vi "HapticSPM_write.vi"() -> ()   [LabVIEW 2021]
uses:
  Haptic-Programming-Interface/LabVIEW VIs/Haptic Prog Interface/Haptic Prog Interface.lvlib
  <userlib>/Nanonis Prog Interface V5/Nanonis Prog Interface.lvlib
panel:
  out "Numeric 3":i32
  out "Numeric 2":i32
  out "Numeric":i32
  in  "Suggested Settings":bool=TRUE
  out "?":bool=TRUE
  out "Surface":dbl caption="Numeric" format="%#_2p"
  out "Z-Position":dbl caption="Numeric" format="%#_2p"
  out "y":string
  out "x":string
  out "scan data":dbl[][](array[numeric])
  out "Force":dbl(slide) scale=-3.0..3.0
  out "Frame String":string
  in  "Stop":bool
  out "Safe tip":bool
  out "Value":dbl caption="Numeric" format="%#_2p"
  out "Reframed Position (m)":cluster{"x (m)":dbl, "y (m)":dbl, "z (m)":dbl} {"z (m)" format="%.1p"; "y (m)" format="%.1p"; "x (m)" format="%.1p"}
  out "Frame Properties (m)":T1
  in  "Function":string(combo)="0" caption="Combo Box"
  in  "Gain (mm/pm)":dbl=1.0 caption="Numeric" format="%.1g"
  in  "k":dbl=1.0 caption="Numeric" step=0.1 format="%.1g"
  in  "Setpoint":dbl=1e-10 caption="Numeric" step=1e-11 format="%.0p"
  in  "Gain":dbl=1.0 caption="Numeric" format="%.1g"
  out "Click Number":dbl caption="Numeric" format="%#_1g"
  in  "Write Z":bool
  in  "Planing Toggle":bool
  in  "Planing Reset":bool
  in  "Save":bool
  # "Super Ultra Mega Haptic SPM Controller 3000"
  # "Scan Window"
  # "Height"
  # "Signal"
  # "Force"
  # "Force"
  # "Planing"
  # "Surface Scale"
  # "Move pens in all three dimensions to calibrate\nClick \"enter\" to turn off recommended settings"
  # "Z Write"
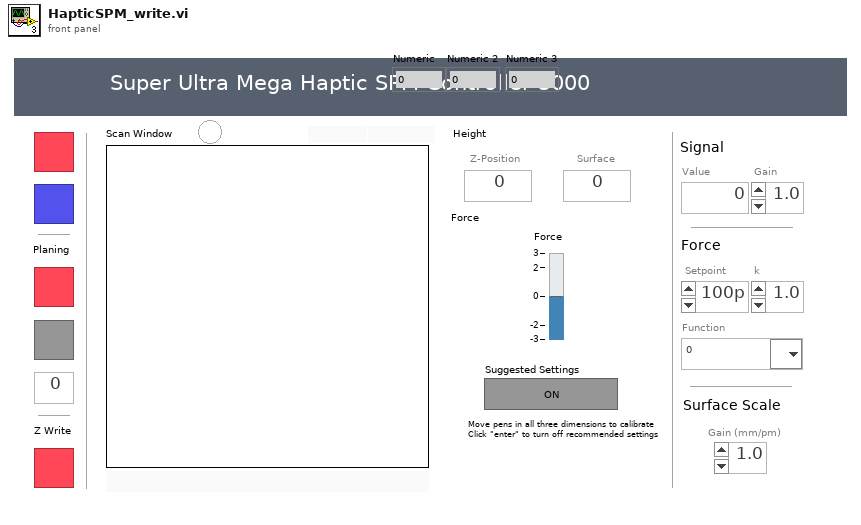
[diagram p1: front panel]
types:
  T1 = cluster{"Center coordinates (m)":cluster{"Xc":sgl, "Yc":sgl}, "Size (m)":cluster{"Width":sgl, "Height":sgl}}
  T2 = cluster{"Fx (N)":dbl, "Fy (N)":dbl, "Fz (N)":dbl}
  T3 = cluster{"kx (N/m)":dbl, "ky (N/m)":dbl, "kz (N/m)":dbl}
  T4 = cluster{"X Drag":bool, "Y Drag":bool, "Z Drag":bool}
  T5 = cluster{"Origin (m)":cluster{"X Origin (m)":dbl, "Y Origin (m)":dbl}, "Frame Size (m)":cluster{"FW (m)":dbl, "FH (m)":dbl}}
  T6 = cluster{"x (mm)":dbl, "y (mm)":dbl, "z (mm)":dbl}
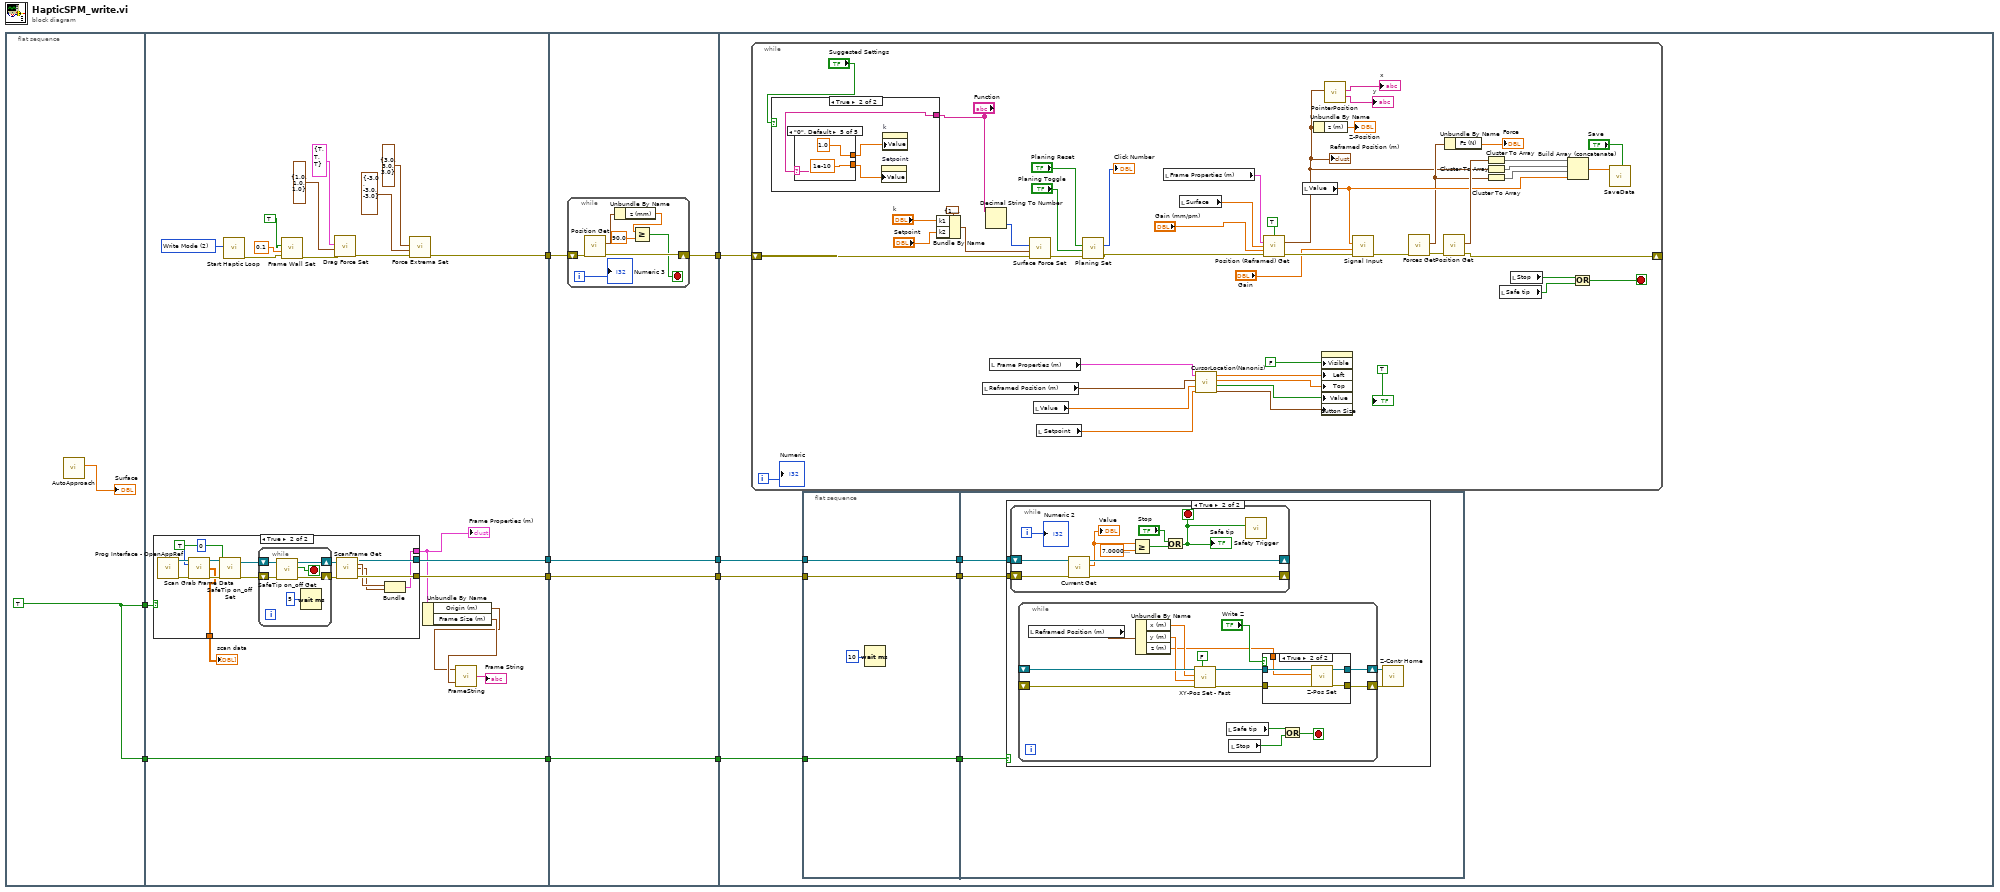
[diagram p0: block diagram]
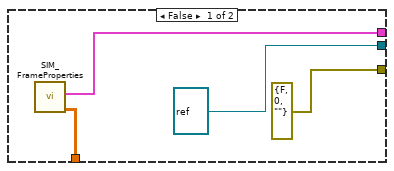
[diagram p2: hidden frame]
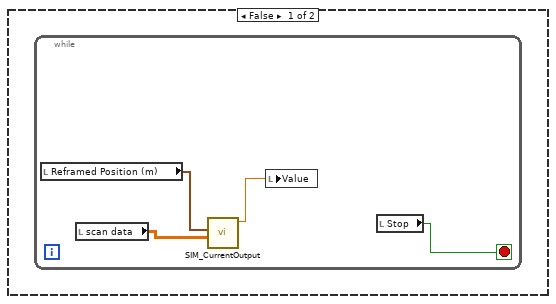
[diagram p3: hidden frame]
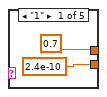
[diagram p6: hidden frame]
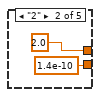
[diagram p7: hidden frame]
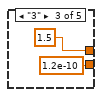
[diagram p8: hidden frame]
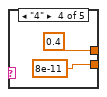
[diagram p9: hidden frame]
diagram:
  n1 = flat-sequence {
    tunnel: [w12] -> w4
    tunnel: [w12] -> w3
    tunnel: [w30] -> w10
    tunnel: [w21] -> w7
    tunnel: [w20] -> w5
    tunnel: w4 -> [w19]
    tunnel: w3 -> [w18]
    tunnel: [w18] -> w2
    tunnel: w10 -> [w63]
    tunnel: [w62] -> w9
    tunnel: [w61] -> w8
    tunnel: w7 -> [w61]
    tunnel: [w60] -> w6
    tunnel: w5 -> [w60]
    tunnel: w2 -> [w59]
    tunnel: [w59] -> w1
    tunnel: w9 -> [w77]
    tunnel: w8 -> [w75]
    tunnel: w6 -> [w73]
    tunnel: w1 -> [w72]
    frame #0 {
      w12 = TRUE
      n2 = call "AutoApproach.vi"() -> ("Surface Location (m)"=→"Surface":dbl)  [unwired: 11 in]
    }
    frame #1 {
      w32 = u16 2 items=["Custom Mode", "Read Mode", "Write Mode"] ("Mode Selection")
      n3 = case shown="True" w19 {
        tunnel: [refnum<vi> refnum ("Application ref out") w47] -> w21
        tunnel: [errorcluster {"status"=FALSE, "code"=0, "source"=""} ("error out") w46] -> w20
        tunnel: [w33 w37] -> w15
        tunnel: [w34 w41] -> w17
        frame False {
          n4 = call "SIM_FrameProperties.vi"() -> ("data"=w34:dbl[][], "Frame Properties (m)"=w33:T5)  [unwired: 9 in, 1 out]
        }
        frame True {
          n5 = call <userlib>:"Prog Interface - OpenAppRef.vi"() -> ("Error out"=w42:errorcluster, "Application reference"=w45:refnum<vi>)  [unwired: 6 in]
          n6 = call <userlib>:"Scan Grab Frame Data.vi"("Application ref in"=w45, "Channel index (0-23)"=u8 0, "error in (no error)"=w42) -> ("Application ref out"=w44:refnum<vi>, "Scan frame data"=w41:sgl[][], "error out"=w43:errorcluster)  [unwired: 8 in, 2 out]
          n7 = call <userlib>:"SafeTip on_off Set.vi"("error in (no error)"=w43, "SafeTip ON/OFF"=TRUE, "Application ref in"=w44) -> ("error out"=w52:errorcluster, "Application ref out"=w51:refnum<vi>)  [unwired: 7 in]
          n8 = while {
            shift-right: [w56] -> w49
            shift-left: w51 -> [w58]
            shift-right: [w55] -> w48
            shift-left: w52 -> [w57]
            stop <- w53 stop-if-true
            n9 = call <userlib>:"SafeTip on_off Get.vi"("error in (no error)"=w57, "Application ref in"=w58) -> ("error out"=w55:errorcluster, "SafeTip on/off status"=w53:bool, "Application ref out"=w56:refnum<vi>)  [unwired: 7 in]
            n10 = Wait (ms)(milliseconds to wait=u32 5) -> ()  [unwired: 1 out]
          }
          n11 = call <userlib>:"ScanFrame Get.vi"("Application ref in"=w49, "error in (no error)"=w48) -> ("Application ref out"=w47:refnum<vi>, "Center coordinates (m)"=w39:cluster{"Xc":sgl, "Yc":sgl}, "Size (m)"=w38:cluster{"Width":sgl, "Height":sgl}, "error out"=w46:errorcluster)  [unwired: 9 in, 1 out]
          n12 = Bundle("Center coordinates (m)"=w39, "Size (m)"=w38) -> (w37:T1)  [unwired: 1 in]
        }
      }
      "Frame Properties (m)" <- w15
      "scan data" <- w17
      n13 = call "Start Haptic Loop.vi"("Mode Selection"=w32) -> ("error out"=w23:errorcluster)  [unwired: 10 in]
      n14 = call "Frame Wall Set.vi"("error in (no error)"=w23, "Wall Stiffness (N/m)"=0.1 ("Wall Stiffness"), "Restrict to Frame"=TRUE) -> ("error out"=w22:errorcluster)  [unwired: 8 in]
      n15 = call "Drag Force Set.vi"("error in (no error)"=w22, "Drag Coefficients (N/m)"=T3 {"kx (N/m)"=1.0, "ky (N/m)"=1.0, "kz (N/m)"=1.0} ("Drag Coefficients"), "Drag Force Toggles"=T4 {"X Drag"=TRUE, "Y Drag"=TRUE, "Z Drag"=TRUE}) -> ("error out"=w31:errorcluster)  [unwired: 8 in]
      n16 = call "Force Extrema Set.vi"("error in (no error)"=w31, "Minimum Force (N)"=T2 {"Fx (N)"=-3.0, "Fy (N)"=-3.0, "Fz (N)"=-3.0} ("Minimum Force"), "Maximum Force (N)"=T2 {"Fx (N)"=3.0, "Fy (N)"=3.0, "Fz (N)"=3.0} ("Maximum Force")) -> ("error out"=w30:errorcluster)  [unwired: 8 in]
      n17 = Unbundle By Name(w15) -> ("Origin (m)"=w13:cluster{"X Origin (m)":dbl, "Y Origin (m)":dbl}, "Frame Size (m)"=w14:cluster{"FW (m)":dbl, "FH (m)":dbl})
      n18 = call "FrameString.vi"("Size (m)"=w14, "Center coordinates (m)"=w13) -> ("string"=→"Frame String":string)
    }
    frame #2 {
      n19 = while {
        shift-right: [w69] -> w62
        shift-left: w63 -> [w70]
        i -> [w64]
        stop <- w65 stop-if-true
        n20 = call "Position Get.vi"("error in (no error)"=w70) -> ("error out"=w69:errorcluster, "Position"=w68:T6)  [unwired: 9 in]
        n21 = Unbundle By Name(w68) -> ("z (mm)"=w67:dbl)
        n22 = Greater Or Equal?(x=w67, y=90.0) -> (x >= y?=w65:bool)
        "Numeric 3" <- w64
      }
    }
    frame #3 {
      n23 = while {
        shift-right: [w166] -> _
        shift-left: w77 -> [w173]
        i -> [w125]
        stop <- w126 stop-if-true
        n24 = case shown="True" "Suggested Settings" {
          tunnel: "Function" -> [_ w176]
          frame False {
          }
          frame True {
            n25 = case shown="\"0\", Default" w176 {
              tunnel: [0.7 2.0 1.5 0.4 1.0] -> w175
              tunnel: [2.4e-10 1.4e-10 1.2e-10 8e-11 1e-10] -> w174
              frame "1" {
              }
              frame "2" {
              }
              frame "3" {
              }
              frame "4" {
              }
              frame "0", Default {
              }
            }
            n26 = property on="Setpoint" class="DigNum (strict)"("Value"=w174) -> ()  [unwired: 2 in, 2 out]
            n27 = property on="k" class="DigNum (strict)"("Value"=w175) -> ()  [unwired: 2 in, 2 out]
          }
        }
        n28 = Bundle By Name(cluster=cluster{"k1":dbl, "k2":dbl, "k3":dbl, "k4":dbl} {"k1"=1.0, "k2"=1.0, "k3"=1.0, "k4"=1.0} ("Force Constants"), "k1"="k", "k2"="Setpoint") -> (w159:cluster{"k1":dbl, "k2":dbl, "k3":dbl, "k4":dbl})
        n29 = local read "Reframed Position (m)"() -> (w129:cluster{"x (m)":dbl, "y (m)":dbl, "z (m)":dbl})
        n30 = Decimal String To Number(string="Function") -> (number=w156:i32)  [unwired: 2 in, 1 out]
        n31 = local read "Frame Properties (m)"() -> (w133:T1)
        n32 = call "Surface Force Set.vi"("error in (no error)"=w173, "Force Constants"=w159, "Force Settings"=w156) -> ("error out"=w172:errorcluster)  [unwired: 8 in]
        n33 = local read "Value"() -> (w132:dbl)
        n34 = local read "Setpoint"() -> (w131:dbl)
        n35 = call "Planing Set.vi"("error in (no error)"=w172, "Planing"="Planing Toggle", "Reset"="Planing Reset") -> ("error out"=w162:errorcluster, "Number of Clicks"=→"Click Number":i8)  [unwired: 7 in]
        n36 = local read "Frame Properties (m)"() -> (w144:T1)
        n37 = local read "Surface"() -> (w170:dbl)
        n38 = call "CursorLocation(Nanonis).vi"("Setpoint"=w131, "Value"=w132, "Position (Reframed)"=w129, "Frame Properties (m)"=w133) -> ("Cursor Size"=w134:cluster{"Width":i32, "Height":i32}, "Current Above Setpoint?"=w135:bool, "Y-Coordinate"=w136:dbl, "X-Coordinate"=w137:dbl)
        n39 = call "Position (Reframed) Get.vi"("Z Rescaling"=TRUE, "Frame Properties (m)"=w144, "Surface Location (m)"=w170, "Scaling (mm per pm)"="Gain (mm/pm)", "error in (no error)"=w162) -> ("Reframed Position (m)"=w140:cluster{"x (m)":dbl, "y (m)":dbl, "z (m)":dbl}, "error out"=w168:errorcluster)  [unwired: 9 in]
        "Reframed Position (m)" <- w140
        n40 = local read "Value"() -> (w150:dbl)
        n41 = Unbundle By Name(w140) -> ("z (m)"=→"Z-Position":dbl)
        n42 = property class="Bool (strict)"("Visible"=FALSE, "Left"=w137, "Top"=w136, "Value"=w135, "Button Size"=w134) -> ()  [unwired: 2 in, 2 out]
        n43 = call "PointerPosition.vi"("Reframed Position (m)"=w140) -> ("y string"=→"y":string, "x string"=→"x":string)  [unwired: 9 in]
        n44 = call "Signal Input.vi"("error in (no error)"=w168, "Gain"="Gain", "Signal"=w150) -> ("error out"=w169:errorcluster)  [unwired: 8 in]
        n45 = call "Forces Get.vi"("error in (no error)"=w169) -> ("error out"=w167:errorcluster, "Force (N)"=w145:T2)  [unwired: 9 in]
        n46 = call "Position Get.vi"("error in (no error)"=w167) -> ("error out"=w166:errorcluster, "Position"=w154:T6)  [unwired: 9 in]
        n47 = Unbundle By Name(w145) -> ("Fz (N)"=→"Force":dbl)
        n48 = Cluster To Array(cluster=w154) -> (array=w153:dbl[])
        n49 = Cluster To Array(cluster=w140) -> (array=w152:dbl[])
        n50 = Cluster To Array(cluster=w145) -> (array=w151:dbl[])
        n51 = local read "Safe tip"() -> (w146:bool)
        n52 = local read "Stop"() -> (w147:bool)
        n53 = Build Array (concatenate)(w153, w152, w151, w150) -> (w149:dbl[])
        n54 = Or(x=w147, y=w146) -> (x .or. y?=w126:bool)
        n55 = call "SaveData.vi"("Save"="Save", "Data"=w149) -> ()  [unwired: 10 in]
        "?" <- TRUE
        "Numeric" <- w125
      }
      n56 = flat-sequence {
        tunnel: [w80] -> w76
        tunnel: w75 -> [w80]
        tunnel: [w79] -> w74
        tunnel: w73 -> [w79]
        tunnel: w72 -> [w78]
        tunnel: [w78] -> w71
        tunnel: w76 -> [w84]
        tunnel: w74 -> [w83]
        tunnel: w71 -> [w82]
        frame #0 {
          n57 = Wait (ms)(milliseconds to wait=u32 10) -> ()  [unwired: 1 out]
        }
        frame #1 {
          n58 = case shown="True" w82 {
            tunnel: w84 -> [_ w92]
            tunnel: w83 -> [_ w91]
            frame False {
              n59 = while {
                stop <- w86 stop-if-true
                n60 = local read "Reframed Position (m)"() -> (w87:cluster{"x (m)":dbl, "y (m)":dbl, "z (m)":dbl})
                n61 = local read "scan data"() -> (w85:dbl[][])
                n62 = call "SIM_CurrentOutput.vi"("array"=w85, "Position (Reframed)"=w87) -> ("Current Out (A)"=w88:dbl)  [unwired: 8 in, 1 out]
                n63 = local write "Value"(w88) -> ()
                n64 = local read "Stop"() -> (w86:bool)
              }
            }
            frame True {
              n65 = while {
                shift-right: [w100] -> _
                shift-left: w92 -> [w102]
                shift-right: [w99] -> _
                shift-left: w91 -> [w101]
                i -> [w93]
                stop <- w94 stop-if-true
                n66 = call <userlib>:"Current Get.vi"("Error in (no error)"=w101, "Application ref in"=w102) -> ("Error out"=w99:errorcluster, "Current (A)"=w98:sgl, "Application ref out"=w100:refnum<vi>)  [unwired: 5 in]
                "Value" <- w98
                n67 = Greater Or Equal?(x=w98, y=sgl 7e-10) -> (x >= y?=w96:bool)
                n68 = Or(x="Stop", y=w96) -> (x .or. y?=w94:bool)
                "Safe tip" <- w94
                n69 = call "Safety Trigger.vi"("Safety Trigger"=w94) -> ()  [unwired: 9 in, 2 out]
                "Numeric 2" <- w93
              }
              n70 = while {
                shift-right: [w110] -> w90
                shift-left: _ -> [w116]
                shift-right: [w108] -> w89
                shift-left: _ -> [w117]
                stop <- w103 stop-if-true
                n71 = local read "Reframed Position (m)"() -> (w115:cluster{"x (m)":dbl, "y (m)":dbl, "z (m)":dbl})
                n72 = Unbundle By Name(w115) -> ("x (m)"=w114:dbl, "y (m)"=w113:dbl, "z (m)"=w106:dbl)
                n73 = call <userlib>:"XY-Pos Set - Fast.vi"("Wait end-of-motion (T=True)"=FALSE, "error in (no error)"=w117, "Y (m)"=w113, "X (m)"=w114, "Application ref in"=w116) -> ("error out"=w107:errorcluster, "Application ref out"=w109:refnum<vi>)  [unwired: 4 in]
                n74 = local read "Safe tip"() -> (w105:bool)
                n75 = local read "Stop"() -> (w104:bool)
                n76 = case shown="True" "Write Z" {
                  tunnel: [w119 w122] -> w110
                  tunnel: w109 -> [w119 w124]
                  tunnel: [w118 w121] -> w108
                  tunnel: w107 -> [w118 w123]
                  tunnel: w106 -> [_ w120]
                  frame False {
                  }
                  frame True {
                    n77 = call <userlib>:"Z-Pos Set.vi"("error in (no error)"=w123, "Z position (m)"=w120, "Application ref in"=w124) -> ("error out"=w121:errorcluster, "Application ref out"=w122:refnum<vi>)  [unwired: 7 in]
                  }
                }
                n78 = Or(x=w105, y=w104) -> (x .or. y?=w103:bool)
              }
              n79 = call <userlib>:"Z-Contr Home.vi"("Error in (no error)"=w89, "Application ref in"=w90) -> ()  [unwired: 8 in, 2 out]
            }
          }
        }
      }
    }
  }
